vi "Save_Log_File.vi"(8 "RX_Station":string="2", 11 "TX_Station":string="1") -> (2 "참조 번호 출력":refnum<file>)   [LabVIEW 2023]
uses:
  <vilib>/Utility/sysdir.llb/System Directory Type.ctl
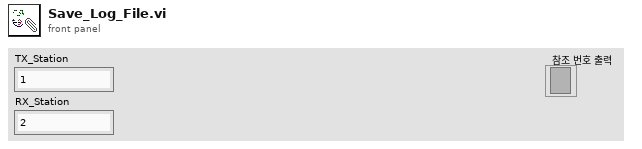
[diagram p1: front panel]
types:
  T1 = enum16{"open", "replace", "create", "open or create", "replace or create", "replace or create with confirmation"}
  T2 = typedef "System Directory Type.ctl" = i32
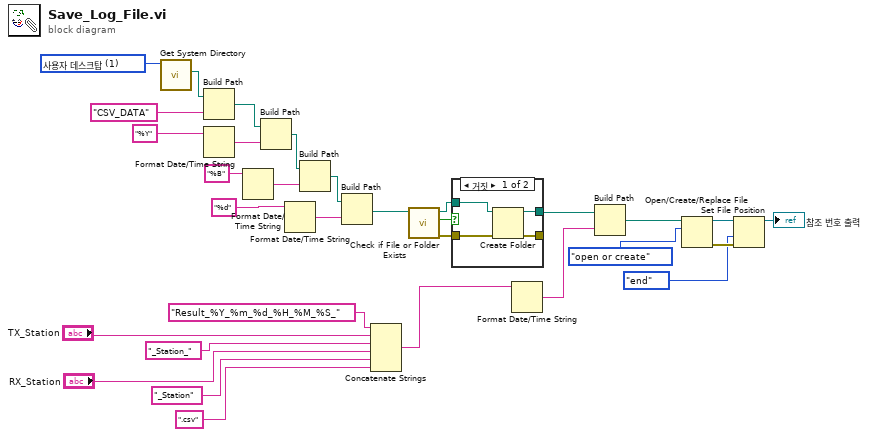
[diagram p0: block diagram]
diagram:
  w25 = T2 1 items=["사용자 홈"=0, "사용자 데스크탑"=1, "사용자 문서"=2, "사용자 어플리케이션 데이터"=3, "사용자 환경"=4, "사용자 임시"=5, "퍼블릭 문서"=6, "퍼블릭 어플리케이션 데이터"=7, "퍼블릭 환경"=8, "퍼블릭 캐시"=13, "시스템 코어 라이브러리"=9, "시스템 설치된 라이브러리"=10, "어플리케이션 파일"=11, "부팅 볼륨 루트"=12] ("system directory type")
  n1 = call <vilib>:"Get System Directory.vi"("system directory type"=w25) -> ("system directory"=w31:path)  [unwired: 10 in]
  n2 = Build Path(base path=w31, name or relative path="CSV_DATA") -> (appended path=w18:path)
  n3 = Format Date/Time String(time format string (%c)="%Y") -> (date/time string=w16:string)  [unwired: 2 in]
  n4 = Format Date/Time String(time format string (%c)="%B") -> (date/time string=w15:string)  [unwired: 2 in]
  n5 = Build Path(base path=w18, name or relative path=w16) -> (appended path=w14:path)
  n6 = Format Date/Time String(time format string (%c)="%d") -> (date/time string=w12:string)  [unwired: 2 in]
  n7 = Build Path(base path=w14, name or relative path=w15) -> (appended path=w11:path)
  n8 = Build Path(base path=w11, name or relative path=w12) -> (appended path=w9:path)
  n9 = Concatenate Strings("Result_%Y_%m_%d_%H_%M_%S_" ("시간 포맷 문자열 (%c)"), "TX_Station", "_Station_" ("시간 포맷 문자열 (%c)"), "RX_Station", "_Station" ("시간 포맷 문자열 (%c)"), ".csv" ("시간 포맷 문자열 (%c)")) -> (w2:string)
  n10 = call <vilib>:"Check if File or Folder Exists.vi"("path"=w9) -> ("error out"=w28:errorcluster, "file or folder exists?"=w30:bool, "dup path"=w29:path)  [unwired: 8 in]
  n11 = case shown="거짓" w30 {
    tunnel: w29 -> [w35 w37]
    tunnel: w28 -> [w34 w36]
    tunnel: [w33 w37] -> w21
    tunnel: [w32 w36] -> _
    frame False {
      n12 = Create Folder(path (use dialog)=w35, error in=w34) -> (created path=w33:path, error out=w32:errorcluster)  [unwired: 1 in, 1 out]
    }
    frame True {
    }
  }
  n13 = Format Date/Time String(time format string (%c)=w2) -> (date/time string=w19:string)  [unwired: 2 in]
  n14 = Build Path(base path=w21, name or relative path=w19) -> (appended path=w20:path)
  n15 = Open/Create/Replace File(file path (use dialog)=w20, operation (0:open)=T1."open or create" ("동작(0:open)")) -> (refnum out=w24:refnum<file>, error out=w23:errorcluster)  [unwired: 4 in, 1 out]
  n16 = Set File Position(refnum=w24, from (0:start)=enum16{"start", "end", "current"}."end" ("위치(0:start)"), error in=w23) -> (refnum out=→"참조 번호 출력":refnum<file>)  [unwired: 1 in, 1 out]
